vi "Multiple Straight Line Moves_simplified.vi"(1 "Target Pulse Duration (ms)":dbl=2.0, 2 "Sync lag":u32=150, 3 "Target Peak Displacement (mm)":dbl=2.0) -> (0 "Single Plot (Array of X,Y Pairs)":cluster{u32[], dbl[]}(graph))   [LabVIEW 2014]
doc: "This example shows a single axis straight-line move using the NI SoftMotion Line function block.\n\nNote: You must have the LabVIEW NI SoftMotion Module installed to run this example."
uses:
  <vilib>/Motion/Express/_s/nimc.fb.straightLineMove.startStraightLineMove.axis.modeRelative.0.vi
  <vilib>/Motion/Express/_s/nimc.fb.stopMove.stop.axis.modeDecelerate.vi
  <vilib>/Motion/Express/_s/nimc.fb.read.readExecutionData.axis.vi
  <vilib>/Motion/BlockNode/FB.NIMotion.xnode
panel:
  out "Expected Pulse Duration":dbl
  out "Acceleration (decimicrons/s2)":dbl
  out "Velocity (decimicrons/s)":dbl
  out "Position at Peak (decimicrons)":dbl
  out "Example Done":bool=TRUE
  out "error out":errorcluster={"status"=FALSE, "code"=77003, "source"="Invoke Node in nimc.fb.straightLineMove.startStraightLineMove.axis.modeAbsolute.0.vi:5060005->Multiple Straight Line Moves.vi"}
  in  "Resource":refnum<k21>="Axis 1"
  # "Computed Inputs"
  # "Target Parameters"
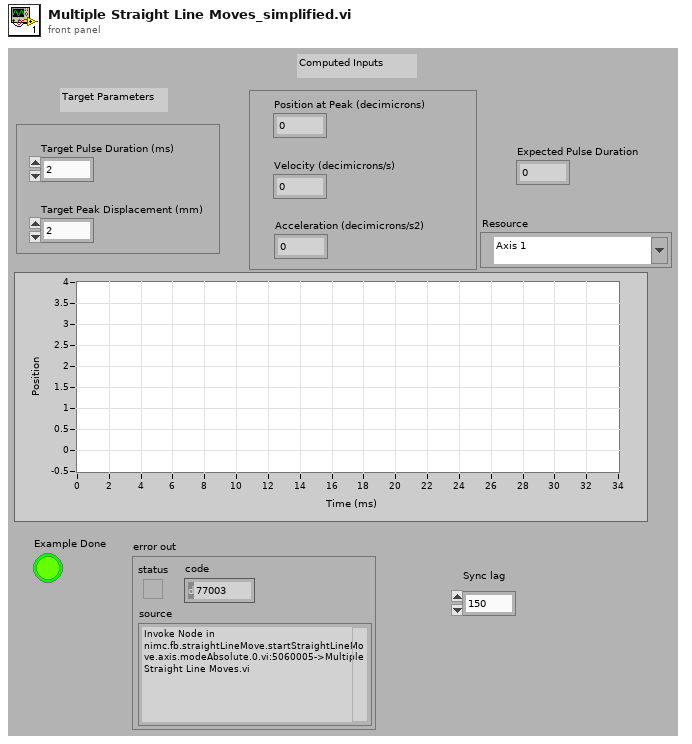
[diagram p1: front panel]
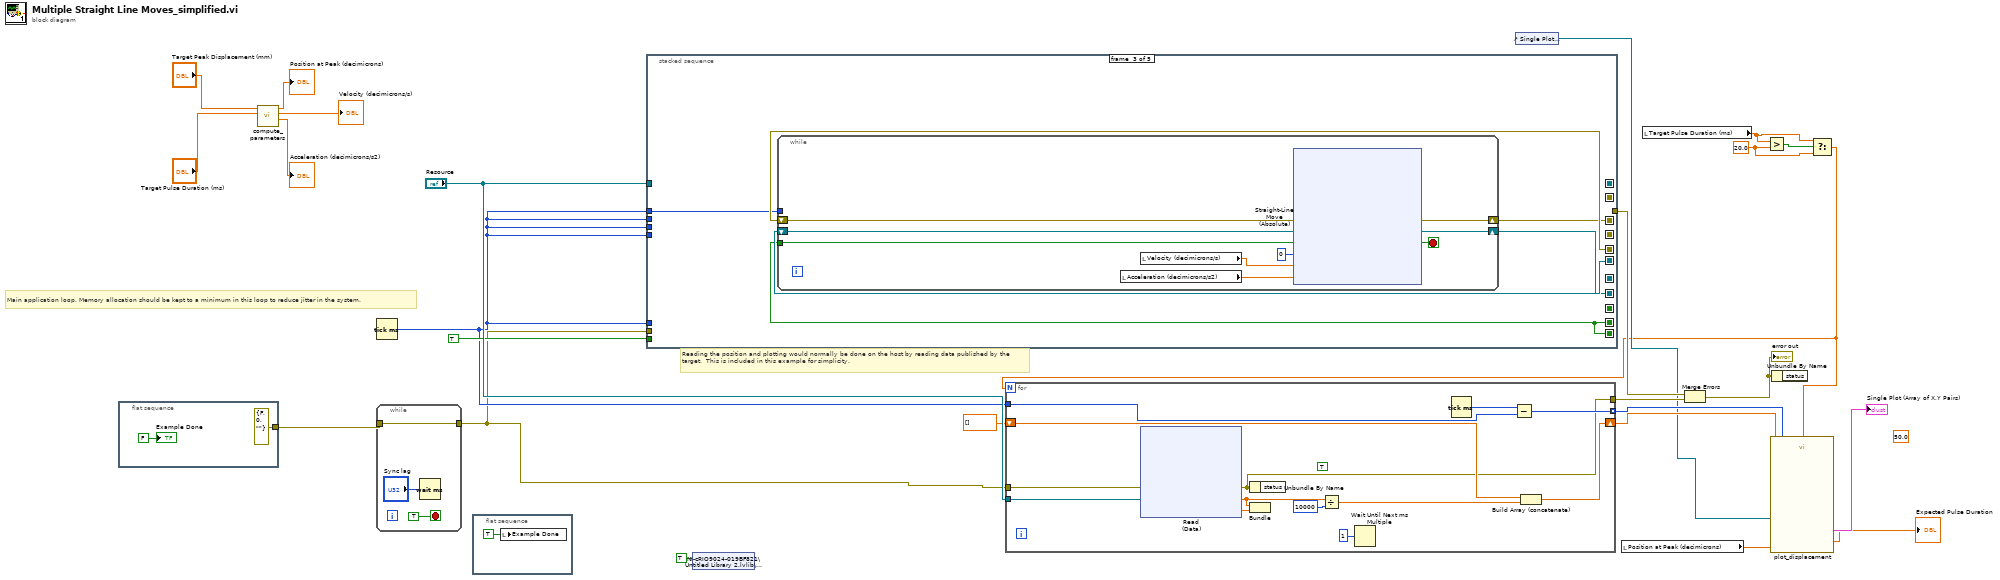
[diagram p0: block diagram]
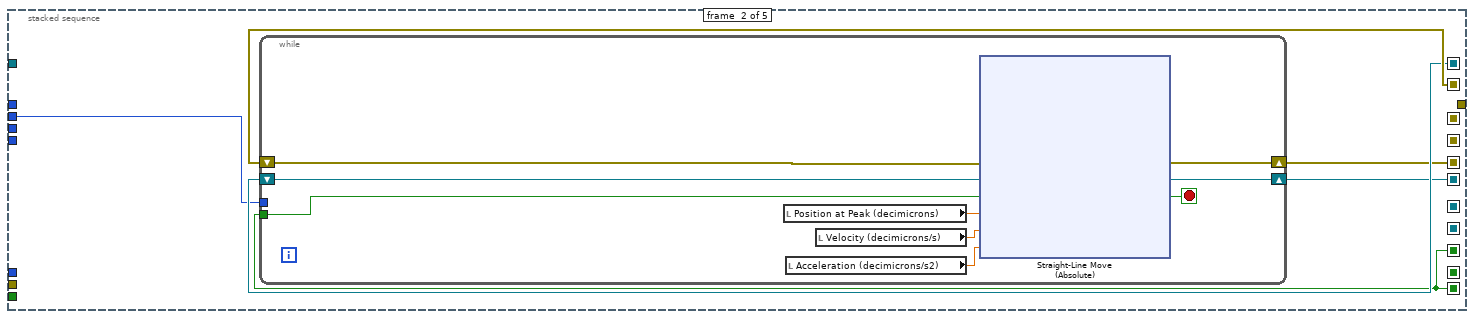
[diagram p3: hidden frame]
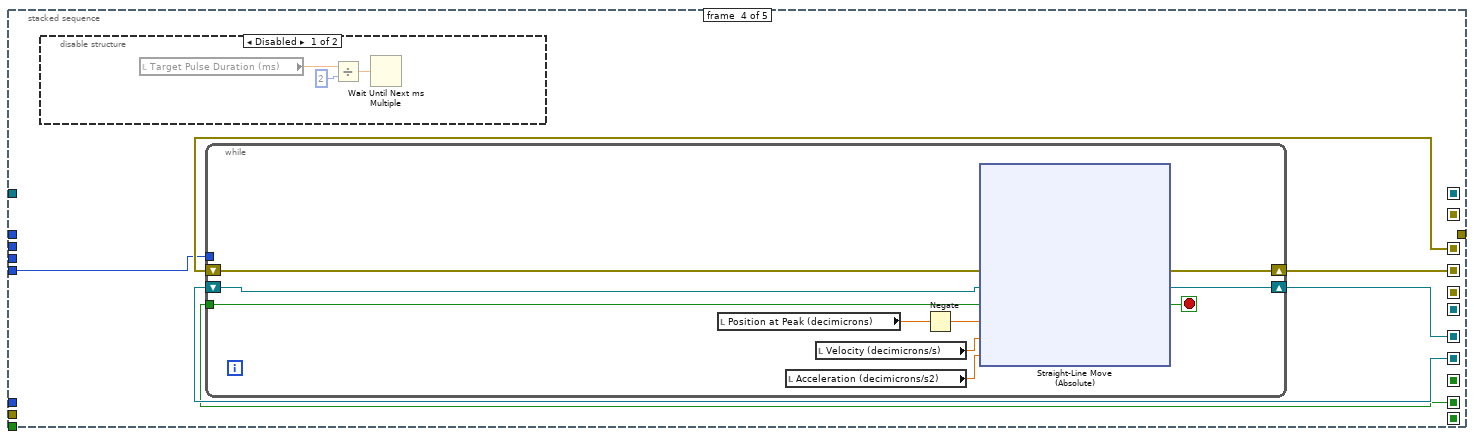
[diagram p4: hidden frame]
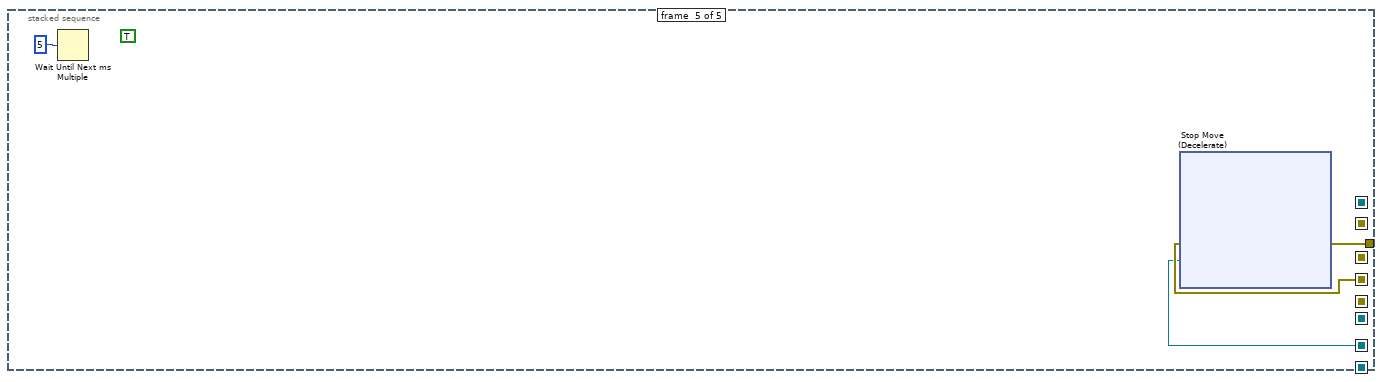
[diagram p6: hidden frame]
diagram:
  (unwired) 50.0 ("X Scale.Range:Maximum")
  w6 = 20.0 ("y")
  # "Reading the position and plotting would normally be done on the host by reading data published by the target.  This is included in this example for simplicity."
  # "Main application loop. Memory allocation should be kept to a minimum in this loop to reduce jitter in the system."
  n1 = flat-sequence {
    tunnel: [errorcluster {"status"=FALSE, "code"=0, "source"=""} ("Error")] -> w2
    frame #0 {
      "Example Done" <- FALSE ("Example Done")
    }
  }
  n2 = call "compute_parameters.vi"("Target Pulse Duration (ms)"="Target Pulse Duration (ms)", "Target Peak Displacement (mm)"="Target Peak Displacement (mm)") -> ("Acceleration (decimicrons/s2)"=→"Acceleration (decimicrons/s2)":dbl, "Velocity (decimicrons/s)"=→"Velocity (decimicrons/s)":dbl, "Position at Peak (decimicrons)"=→"Position at Peak (decimicrons)":dbl)  [unwired: 7 in]
  n3 = Tick Count (ms)() -> (millisecond timer value=w21:u32)
  n4 = while {
    tunnel: [w28] -> w9
    tunnel: w2 -> [w28]
    stop <- TRUE stop-if-true
    n5 = Wait (ms)(milliseconds to wait="Sync lag") -> ()  [unwired: 1 out]
  }
  n6 = flat-sequence {
    frame #0 {
      n7 = local write "Example Done"(TRUE ("Example Done")) -> ()
    }
  }
  n8 = stacked-sequence {
    seq-local: [w32 _ _ _ _] -> [_ w40 _ _ _]
    seq-local: [w33 _ _ _ _] -> [_ w39 _ _ _]
    seq-local: [w34 _ _ _ _] -> [_ w36 _ _ _]
    seq-local: [_ w38 _ _ _] -> [_ _ w72 _ _]
    seq-local: [_ w37 _ _ _] -> [_ _ w70 _ _]
    seq-local: [_ w36 _ _ _] -> [_ _ w68 _ _]
    seq-local: [_ _ w71 _ _] -> [_ _ _ w104 _]
    seq-local: [_ _ w69 _ _] -> [_ _ _ w102 _]
    seq-local: [_ _ w68 _ _] -> [_ _ _ w100 _]
    seq-local: [_ _ _ w103 _] -> [_ _ _ _ w138]
    seq-local: [_ _ _ w101 _] -> [_ _ _ _ w136]
    tunnel: "Resource" -> [w33 _ _ _ _]
    tunnel: w9 -> [w32 _ _ _ _]
    tunnel: TRUE ("approach forward") -> [w34 _ _ _ _]
    tunnel: w21 -> [_ _ _ _ _]
    tunnel: w21 -> [_ w35 _ _ _]
    tunnel: w21 -> [_ _ w67 _ _]
    tunnel: w21 -> [_ _ _ w99 _]
    tunnel: [_ _ _ _ w137] -> w22
    tunnel: w21 -> [_ _ _ _ _]
    frame #0 {
    }
    frame #1 {
      n9 = while {
        tunnel: w36 -> [w46]
        tunnel: w35 -> [_]
        shift-right: [w48] -> w38
        shift-left: w40 -> [w41]
        shift-right: [w47] -> w37
        shift-left: w39 -> [w49]
        stop <- w42 stop-if-true
        n10 = local read "Position at Peak (decimicrons)"() -> (w45:dbl)
        n11 = local read "Acceleration (decimicrons/s2)"() -> (w43:dbl)
        n12 = local read "Velocity (decimicrons/s)"() -> (w44:dbl)
        n13 = xnode "Straight-Line Move\n(Absolute)"("error in"=w41, "resource"=w49, "execute"=w46, "position"=w45, "velocity"=w44, "acceleration"=w43) -> ("error out"=w48:errorcluster, "resource out"=w47:refnum<k21>, "done"=w42:bool)
      }
    }
    frame #2 {
      n14 = while {
        tunnel: w68 -> [w77]
        tunnel: w67 -> [_]
        shift-right: [w80] -> w71
        shift-left: w72 -> [w81]
        shift-right: [w78] -> w69
        shift-left: w70 -> [w79]
        stop <- w73 stop-if-true
        n15 = local read "Acceleration (decimicrons/s2)"() -> (w75:dbl)
        n16 = local read "Velocity (decimicrons/s)"() -> (w76:dbl)
        n17 = xnode "Straight-Line Move\n(Absolute)"("error in"=w81, "resource"=w79, "execute"=w77, "position"=0, "velocity"=w76, "acceleration"=w75) -> ("error out"=w80:errorcluster, "resource out"=w78:refnum<k21>, "done"=w73:bool)
      }
    }
    frame #3 {
      n18 = disable-structure shown="Disabled" {
        frame Disabled {
          n19 = local read "Target Pulse Duration (ms)"() -> (w105:dbl)
          n20 = Divide(x=w105, y=2) -> (x/y=w106:dbl)
          n21 = Wait Until Next ms Multiple(millisecond multiple=w106) -> ()  [unwired: 1 out]
        }
        frame Enabled {
        }
      }
      n22 = while {
        tunnel: w100 -> [w113]
        tunnel: w99 -> [_]
        shift-right: [w116] -> w103
        shift-left: w104 -> [w117]
        shift-right: [w114] -> w101
        shift-left: w102 -> [w115]
        stop <- w108 stop-if-true
        n23 = local read "Position at Peak (decimicrons)"() -> (w110:dbl)
        n24 = local read "Acceleration (decimicrons/s2)"() -> (w111:dbl)
        n25 = local read "Velocity (decimicrons/s)"() -> (w112:dbl)
        n26 = Negate(x=w110) -> (-x=w109:dbl)
        n27 = xnode "Straight-Line Move\n(Absolute)"("error in"=w117, "resource"=w115, "execute"=w113, "position"=w109, "velocity"=w112, "acceleration"=w111) -> ("error out"=w116:errorcluster, "resource out"=w114:refnum<k21>, "done"=w108:bool)
      }
    }
    frame #4 {
      (unwired) TRUE
      n28 = Wait Until Next ms Multiple(millisecond multiple=u32 5) -> ()  [unwired: 1 out]
      n29 = xnode "Stop Move\n(Decelerate)"("error in"=w138, "resource"=w136) -> ("error out"=w137:errorcluster)  [unwired: 1 in, 1 out]
    }
  }
  n30 = shared-variable "NI-cRIO9024-019BF821\\Untitled Library 2.lvlib\\Variable2"(TRUE ("Variable2")) -> ()  [unwired: 1 in, 1 out]
  n31 = control-ref of="Single Plot (Array of X,Y Pairs)"() -> (w10:refnum<vi>)
  n32 = local read "Position at Peak (decimicrons)"() -> (w13:dbl)
  n33 = local read "Target Pulse Duration (ms)"() -> (w7:dbl)
  n34 = Greater?(x=w7, y=w6) -> (0:w8:bool)
  n35 = Select(t=w7, s=w8, f=w6) -> (s? t:f=w3:dbl)
  n36 = for {
    N: w3 -> [_]
    tunnel: "Resource" -> [w157]
    tunnel: w9 -> [w158]
    tunnel: [w146] -> w24
    tunnel: w21 -> [w154]
    shift-right: [w150] -> w12
    shift-left: dbl[] [] -> [w151]
    tunnel: [w147] -> w11 mode=indexing
    (unwired) TRUE ("Variable2")
    n37 = xnode "Read\n(Data)"("error in"=w158, "resource"=w157) -> ("error out"=w146:errorcluster, "position"=w152:dbl, "velocity"=w156:dbl)
    n38 = Unbundle By Name(w146) -> ()  [unwired: 1 out]
    n39 = Bundle("position"=w152, "velocity"=w156) -> ()  [unwired: 2 out]
    n40 = Divide(x=w152, y=10000) -> (x/y=w149:dbl)
    n41 = Wait Until Next ms Multiple(millisecond multiple=u32 1) -> ()  [unwired: 1 out]
    n42 = Tick Count (ms)() -> (millisecond timer value=w155:u32)
    n43 = Subtract(x=w155, y=w154) -> (x-y=w147:u32)
    n44 = Build Array (concatenate)(w151, w149) -> (w150:dbl[])
  }
  n45 = Merge Errors(w22, w24) -> (w4:errorcluster)
  "error out" <- w4
  n46 = call "plot_displacement.vi"("Position at Peak (decimicrons)"=w13, "Target Pulse Duration (ms)"=w3, "Array"=w12, "Array 2"=w11, "XYGraph in"=w10) -> ("true pulse duration"=→"Expected Pulse Duration":dbl, "Cluster"=→"Single Plot (Array of X,Y Pairs)":cluster{u32[], dbl[]})  [unwired: 5 in]
  n47 = Unbundle By Name(w4) -> ()  [unwired: 1 out]
